vi "subFixPathSeparatorOnWindows.vi"(11 "Value":string) -> (3 "fixed path":string)   [LabVIEW 2019, in "SolutionBuilder.lvlib" / "SolutionBuilder.lvclass"]
uses:
  SolutionBuilder.lvclass
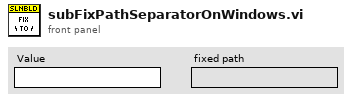
[diagram p1: front panel]
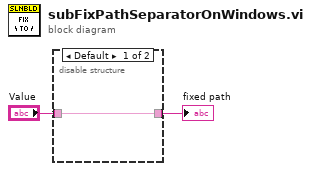
[diagram p0: block diagram]
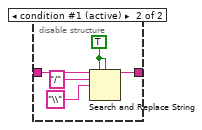
[diagram p2: hidden frame]
diagram:
  n1 = disable-structure shown="Default" {
    disable-tunnel: [w3 w8] -> w2
    disable-tunnel: "Value" -> [w3 w7]
    frame condition #0 {
    }
    frame condition #1 (active) {
      w6 = TRUE ("replace all? (F)")
      n2 = Search and Replace String(replace all?=w6, case sensitive?=w6, input string=w7, search string="/", replace string="\\" ("replace string (\"\")")) -> (result string=w8:string)  [unwired: 3 in, 3 out]
    }
  }
  "fixed path" <- w2
